vi "Set JSON CFG.vi"(10 "<JSON>Data SInk CFG":string, 11 "IData Sink in":refnum<class "IData Sink.lvclass">) -> (3 "IData Sink out":refnum<class "IData Sink.lvclass">)   [LabVIEW 2023, in "IData Sink.lvclass"]
uses:
  IData Sink.lvclass
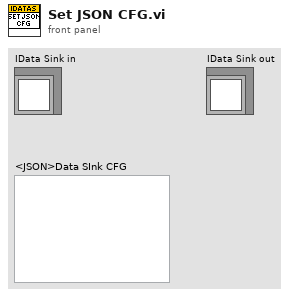
[diagram p1: front panel]
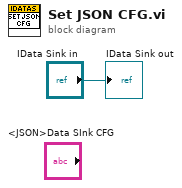
[diagram p0: block diagram]
diagram:
  "IData Sink out" <- "IData Sink in"
